vi "Capacitance_IS_Measure.vi"() -> ()   [LabVIEW 2023, in "Capacitance.lvlib"]
uses:
  Capacitance.lvlib
  <vilib>/NI_TestStand_SemiconductorModule/NI_TestStand_Semiconductor_Module.lvlibp
  <vilib>/NI_TestStand_SemiconductorModule/NI_TestStand_Semiconductor_Module.lvlibp/PinMap/DC Power/PinsToNIDCPowerSessions.vi
  <vilib>/NI_TestStand_SemiconductorModule/NI_TestStand_Semiconductor_Module.lvlibp/PinMap/FGEN/PinsToNIFGenSessions.vi
  <vilib>/NI_TestStand_SemiconductorModule/NI_TestStand_Semiconductor_Module.lvlibp/PinMap/Scope/PinsToNISCOPESessions.vi
  <vilib>/NI_TestStand_SemiconductorModule/NI_TestStand_Semiconductor_Module.lvlibp/PinMap/Scope/PinsToNISCOPESession.vi
  <instrlib>/niScope/Acquire/Fetch/niScope Multi Fetch WDT.vi
  <vilib>/Analysis/NI_AALPro.lvlib
  <vilib>/Analysis/2dsp.llb/Real FFT.vi
  <vilib>/NI_TestStand_SemiconductorModule/NI_TestStand_Semiconductor_Module.lvlibp/PinMap/General/SemiconductorModuleContext.ctl
  <vilib>/NI_TestStand_SemiconductorModule/NI_TestStand_Semiconductor_Module.lvlibp/PinMap/TagProvider/TSM_Pin.ctl
panel:
  in  "FGEN Pins":T1[](array[typedef])
  in  "SCOPE Pins":T1[](array[typedef])
  in  "DCPower Pins":T1[](array[typedef])
  in  "Semiconductor Module Context":T2
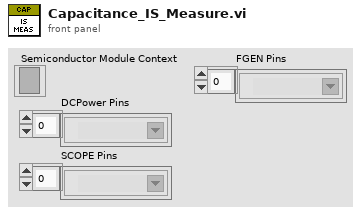
[diagram p1: front panel]
types:
  T1 = typedef "NI_TestStand_Semiconductor_Module.lvlibp/TSM_Pin.ctl" = tag
  T2 = typedef "NI_TestStand_Semiconductor_Module.lvlibp/SemiconductorModuleContext.ctl" = refnum<k7>
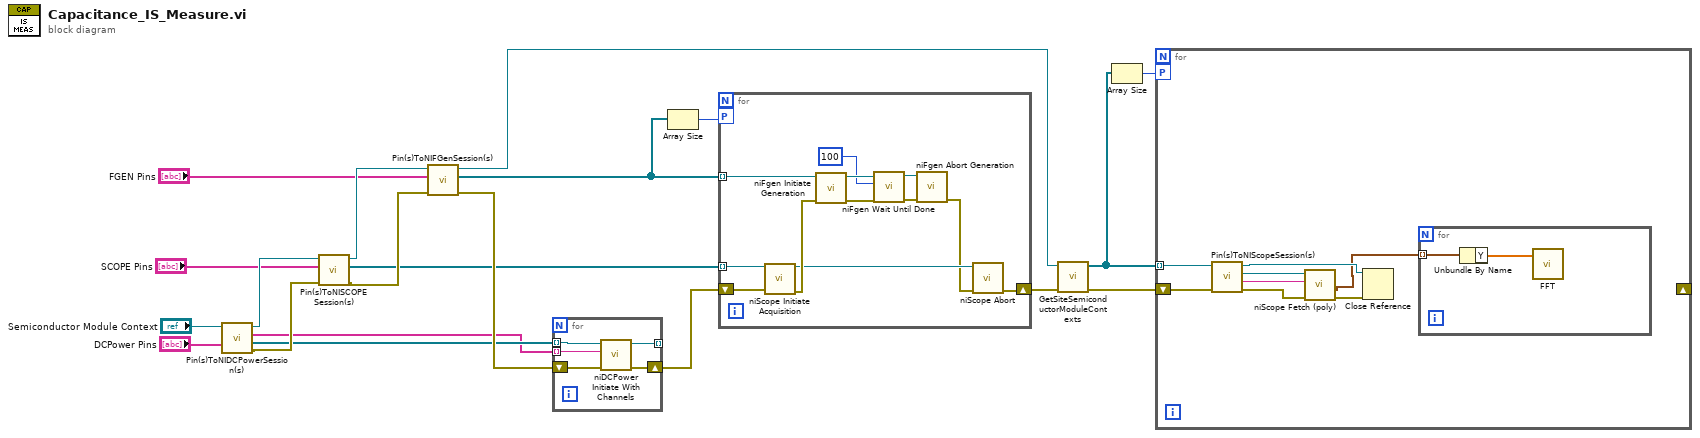
[diagram p0: block diagram]
diagram:
  n1 = call-poly <vilib>:"Pin(s)ToNIDCPowerSession(s).vi"("Pins"="DCPower Pins", "Semiconductor Module Context"="Semiconductor Module Context") -> ("error out"=w18:errorcluster, "Instrument Sessions"=w11:refnum<k15>[], "Channel Strings"=w10:string[], "Semiconductor Module Context Out"=w19:T2)  [unwired: 5 in, 1 out]
  n2 = call-poly <vilib>:"Pin(s)ToNISCOPESession(s).vi"("error in (no error)"=w18, "Pins"="SCOPE Pins", "Semiconductor Module Context"=w19) -> ("error out"=w17:errorcluster, "Instrument Sessions"=w8:refnum<k15>[], "Semiconductor Module Context Out"=w16:T2)  [unwired: 4 in, 2 out]
  n3 = call-poly <vilib>:"Pin(s)ToNIFGenSession(s).vi"("error in (no error)"=w17, "Pins"="FGEN Pins", "Semiconductor Module Context"=w16) -> ("error out"=w12:errorcluster, "Instrument Sessions"=w7:refnum<k15>[], "Semiconductor Module Context Out"=w5:T2)  [unwired: 4 in, 2 out]
  n4 = for {
    shift-right: [w22] -> w9
    shift-left: w12 -> [w25]
    tunnel: w11 -> [w23] mode=indexing
    tunnel: w10 -> [w24] mode=indexing
    tunnel: [w21] -> _ mode=indexing
    n5 = call <instrlib>:"niDCPower Initiate With Channels.vi"("error in (no error)"=w25, "channel name"=w24, "instrument handle"=w23) -> ("error out"=w22:errorcluster, "instrument handle out"=w21:refnum<k15>)  [unwired: 7 in]
  }
  n6 = Array Size(array=w7) -> (size(s)=w6:i32)
  n7 = for {
    shift-right: [w26] -> w4
    shift-left: w9 -> [w36]
    tunnel: w7 -> [w35] mode=indexing
    tunnel: w8 -> [w37] mode=indexing
    workers-P: w6 -> [_]
    n8 = call <instrlib>:"niScope Initiate Acquisition.vi"("instrument handle"=w37, "error in"=w36) -> ("instrument handle out"=w28:refnum<k15>, "error out"=w34:errorcluster)  [unwired: 12 in]
    n9 = call <instrlib>:"niFgen Initiate Generation.vi"("error in (no error)"=w34, "Instrument Handle"=w35) -> ("error out"=w32:errorcluster, "Instrument Handle Out"=w33:refnum<k15>)  [unwired: 8 in]
    n10 = call <instrlib>:"niFgen Wait Until Done.vi"("error in (no error)"=w32, "MaxTime (msec)"=100, "Instrument Handle"=w33) -> ("error out"=w29:errorcluster, "Instrument Handle Out"=w30:refnum<k15>)  [unwired: 7 in]
    n11 = call <instrlib>:"niFgen Abort Generation.vi"("error in (no error)"=w29, "Instrument Handle"=w30) -> ("error out"=w27:errorcluster)  [unwired: 8 in, 1 out]
    n12 = call <instrlib>:"niScope Abort.vi"("instrument handle"=w28, "error in"=w27) -> ("error out"=w26:errorcluster)  [unwired: 12 in, 1 out]
  }
  n13 = call <vilib>:"GetSiteSemiconductorModuleContexts.vi"("error in (no error)"=w4, "Semiconductor Module Context"=w5) -> ("error out"=w3:errorcluster, "Site Semiconductor Module Contexts"=w1:T2[])  [unwired: 8 in]
  n14 = Array Size(array=w1) -> (size(s)=w2:i32)
  n15 = for {
    tunnel: w1 -> [w44] mode=indexing
    shift-right: _ -> [_]
    shift-left: w3 -> [w45]
    workers-P: w2 -> [_]
    n16 = call-poly <vilib>:"Pin(s)ToNIScopeSession(s).vi"("error in (no error)"=w45, "Semiconductor Module Context"=w44) -> ("error out"=w42:errorcluster, "Channel List"=w41:string, "Instrument Session"=w43:refnum<k15>, "Semiconductor Module Context Out"=w39:T2)  [unwired: 5 in, 1 out]
    n17 = call-poly <instrlib>:"niScope Fetch (poly).vi"("error in"=w42, "channels"=w41, "instrument handle"=w43) -> ("error out"=w40:errorcluster, "wfm"=w38:waveform(dbl)[])  [unwired: 5 in, 2 out]
    n18 = Close Reference(reference=w39, error in (no error)=w40) -> ()  [unwired: 1 out]
    n19 = for {
      tunnel: w38 -> [w47] mode=indexing
      n20 = Unbundle By Name(w47) -> ("Y"=w46:dbl[])
      n21 = call-poly <vilib>:"FFT.vi"("X"=w46) -> ()  [unwired: 9 in, 2 out]
    }
  }
